vi "Handle Click on Tree Item.vi"(5 "Button":u16, 7 "PlatMods":T1, 8 "error in (no error)":errorcluster, 9 "Mods":cluster{"Double Click":bool, "Menu Key":bool}, 10 "Coords":T2, 11 "Process Explorer View in":refnum<class "Process Explorer View.lvclass">) -> (0 "error out":errorcluster, 3 "Process Explorer View out":refnum<class "Process Explorer View.lvclass">)   [LabVIEW 2019, in "Process Explorer View.lvclass"]
doc: "<RequiredOverrideReason>Implement the response to the user left clicking on the tree.</RequiredOverrideReason>"
uses:
  <vilib>/gpm_packages/@cs/Car-wash/Source/Process Explorer View/Process Explorer View.lvclass
  <vilib>/gpm_packages/@cs/file-explorer-extension/Source/File Explorer/File Explorer/File Explorer.lvclass
  C:/Program Files/National Instruments/LabVIEW 2019/vi.lib/gpm_packages/@cs/file-explorer-extension/Source/File Explorer/File Explorer/File Explorer.lvclass
  C:/Program Files/National Instruments/LabVIEW 2019/vi.lib/gpm_packages/@cs/mva-viewable/Source/IViewable/IViewable/IViewable.lvclass
  C:/Program Files/National Instruments/LabVIEW 2019/vi.lib/gpm_packages/@cs/mva-viewable/Source/ActorEvents/IEventAggregator/IEventAggregator.lvclass
  C:/Program Files/National Instruments/LabVIEW 2019/vi.lib/gpm_packages/@cs/mva-core/Source/IObserver/IObserver/IObserver.lvclass
  C:/Program Files/National Instruments/LabVIEW 2019/vi.lib/ActorFramework/Actor/Actor.lvclass
  <vilib>/Utility/miscctls.llb/LVPoint32TypeDef.ctl
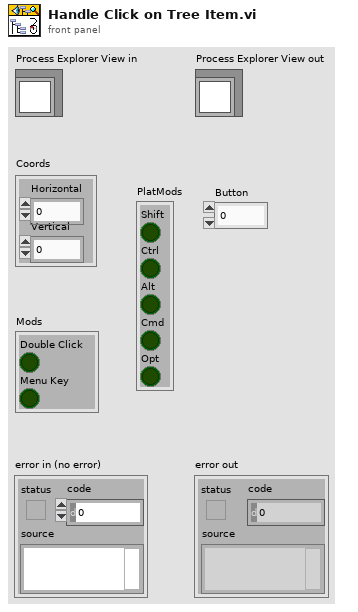
[diagram p1: front panel]
types:
  T1 = cluster{"Shift":bool, "Ctrl":bool, "Alt":bool, "Cmd":bool, "Opt":bool}
  T2 = typedef "LVPoint32TypeDef.ctl" = cluster{"Horizontal":i32, "Vertical":i32}
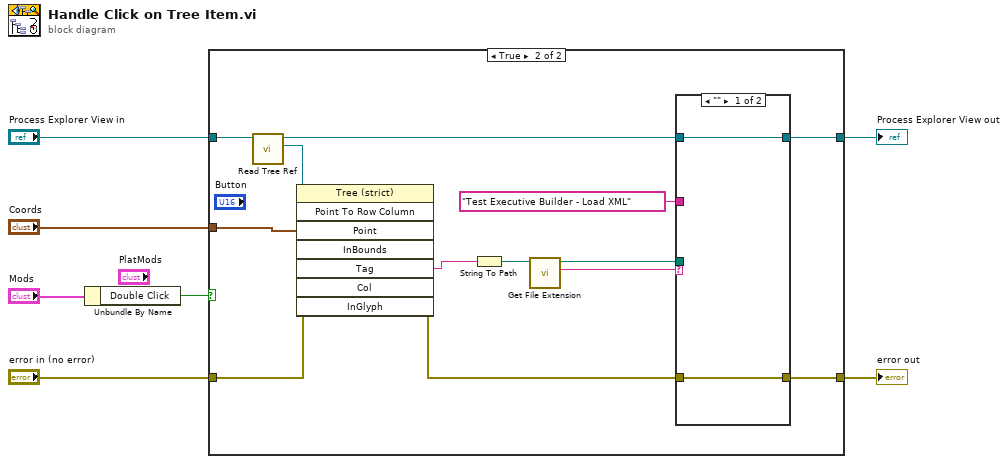
[diagram p0: block diagram]
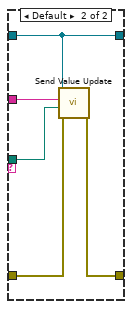
[diagram p3: hidden frame]
diagram:
  n1 = Unbundle By Name("Mods") -> ("Double Click"=w7:bool)
  n2 = case shown="True" w7 {
    tunnel: "Process Explorer View in" -> [w9 w14]
    tunnel: [w9 w13] -> w6
    tunnel: "error in (no error)" -> [w8 w12]
    tunnel: [w8 w11] -> w1
    tunnel: "Coords" -> [_ w10]
    frame False {
    }
    frame True {
      n3 = call <vilib>:"Read Tree Ref.vi"("File Explorer in"=w14) -> ("Tree Ref"=w22:refnum<vi>, "File Explorer out"=w21:refnum<class "Process Explorer View.lvclass">)  [unwired: 8 in, 1 out]
      n4 = invoke class="Tree (strict)" method="Point To Row Column"(reference=w22, error in=w12, "Point"=w10) -> (error out=w18:errorcluster, "Tag"=w16:string)  [unwired: 5 in, 6 out]
      n5 = String To Path(string=w16) -> (path=w20:path)
      n6 = call <vilib>:"Get File Extension.vi"("file"=w20) -> ("lowercase file extension"=w15:string, "dup file"=w17:path)  [unwired: 6 in, 3 out]
      n7 = case shown="\"\"" w15 {
        tunnel: w21 -> [w23 w25]
        tunnel: "Test Executive Builder - Load XML" ("Datum Name") -> [_ w29]
        tunnel: w18 -> [w24 w28]
        tunnel: [w24 w27] -> w11
        tunnel: w17 -> [_ w26]
        tunnel: [w23 w25] -> w13
        frame "" {
        }
        frame Default {
          n8 = call-dynamic "Send Value Update.vi"("error in (no error)"=w28, "Value"=w26, "Datum Name"=w29, "IViewable in"=w25) -> ("error out"=w27:errorcluster)  [unwired: 7 in]
        }
      }
    }
  }
  "error out" <- w1
  "Process Explorer View out" <- w6
